vi "update.vi"(8 "error in (no error)":errorcluster, 11 "HSDIO in":refnum<class "HSDIO.lvclass">) -> (0 "error out":errorcluster, 3 "HSDIO out":refnum<class "HSDIO.lvclass">)   [LabVIEW 2013, in "HSDIO.lvclass"]
uses:
  HSDIO.lvclass
  waveform.ctl
  HSDIO.lvclass/HSDIO.ctl
  Globals.vi
  <instrlib>/niHSDIO/niHSDIO.llb/niHSDIO Write Named Waveform (WDT).vi
panel:
  out "transitions":u32[](array[numeric])
  out "states":u8[][](array[numeric])
  out "output waveform":digitaldata
  out "HSDIO Settings.Array of Waveforms":T1[](array[typedef])
  out "HSDIO Settings.Pulse Generation Script":string
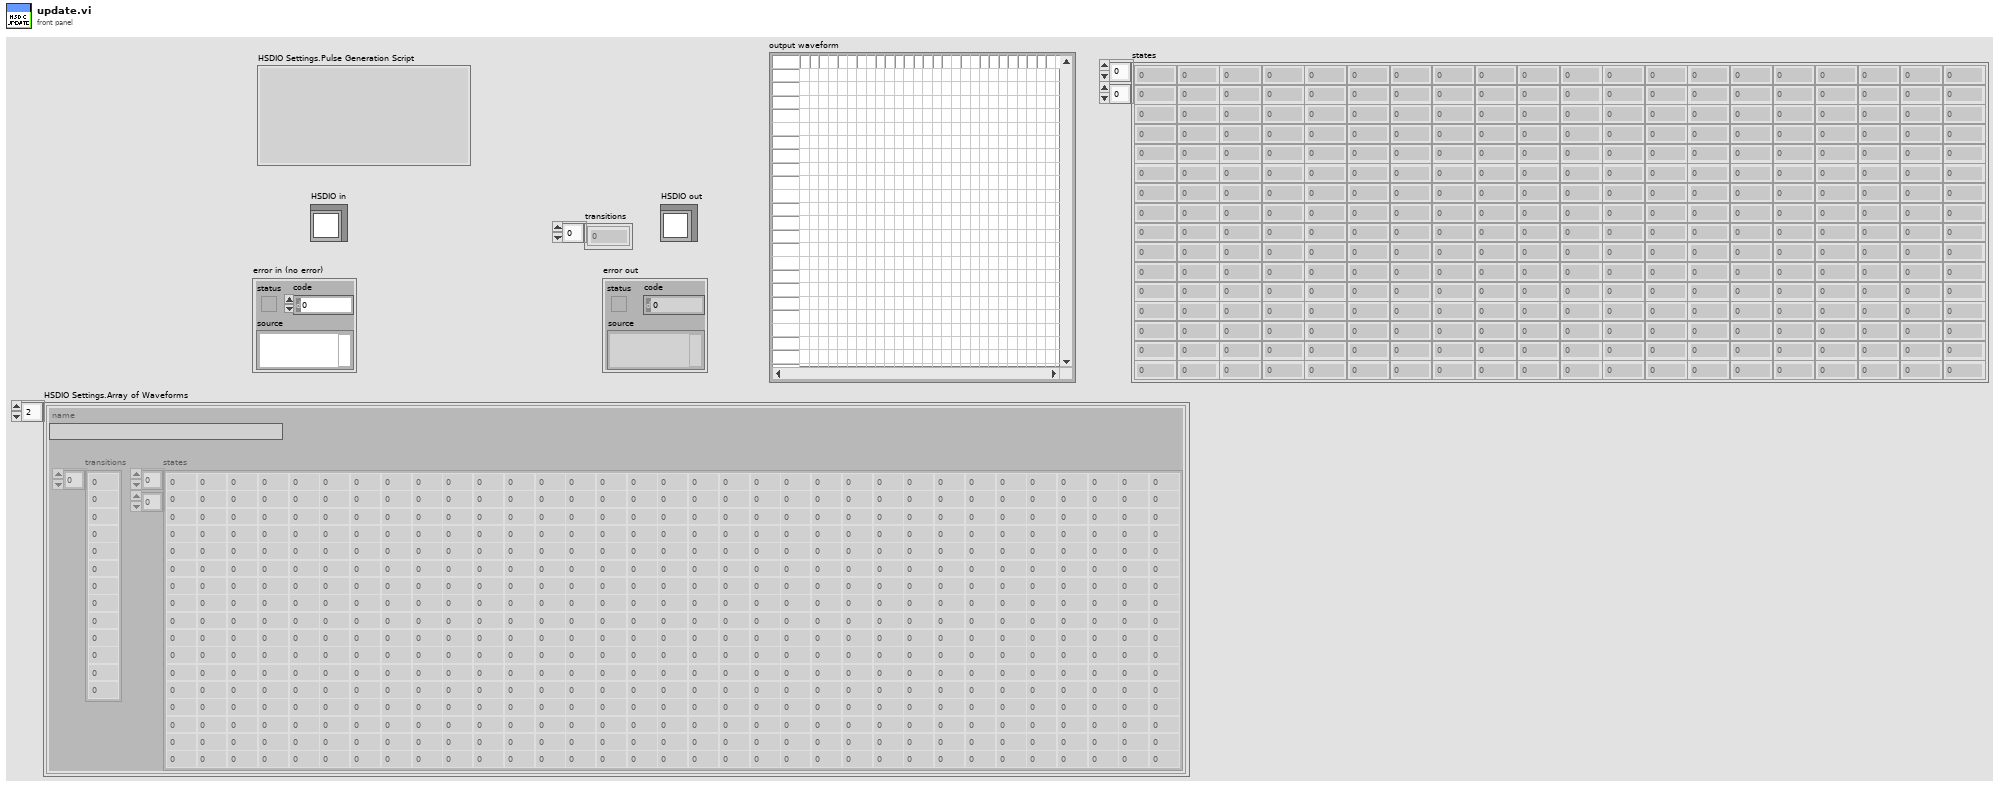
[diagram p1: front panel]
types:
  T1 = typedef "HSDIO.lvclass/waveform.ctl" = cluster{"name":string, "transitions":u32[], "states":u8[][]}
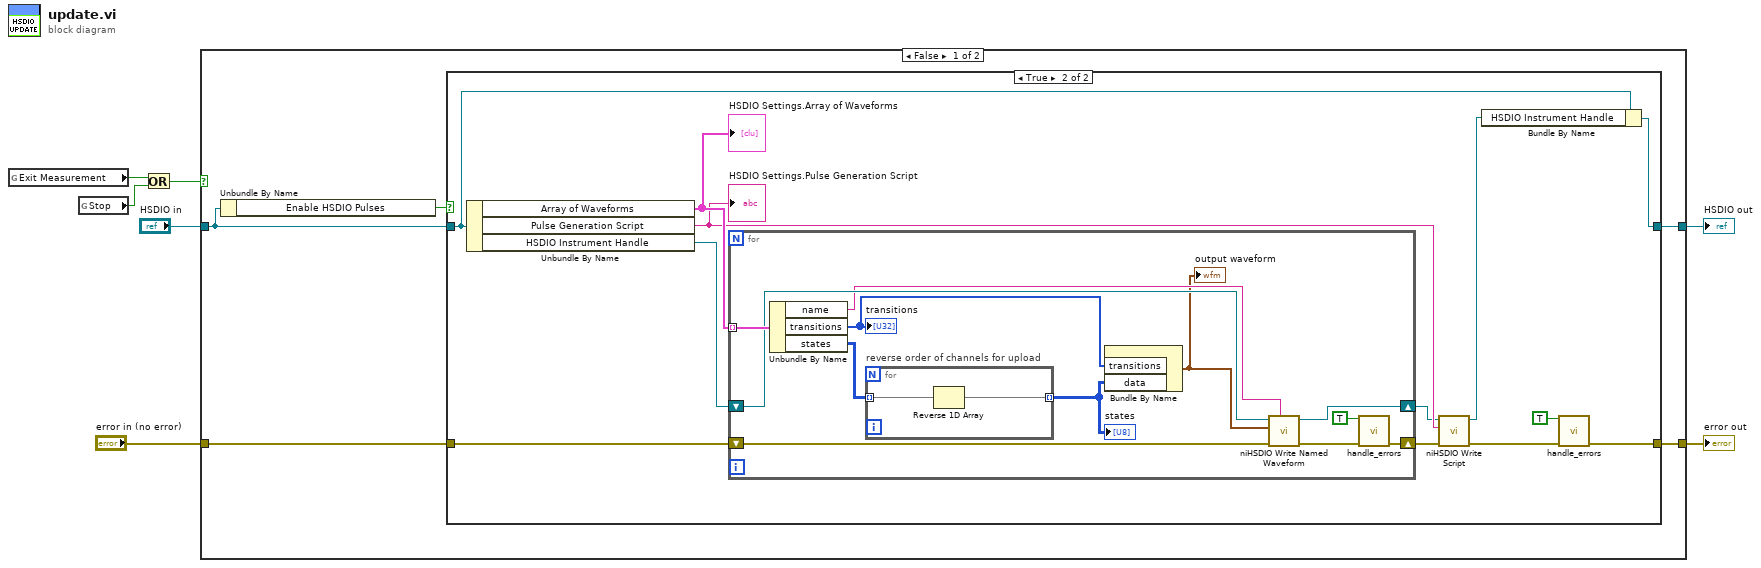
[diagram p0: block diagram]
diagram:
  n1 = global read "Globals.vi" "Exit Measurement"() -> (w3:bool)
  n2 = global read "Globals.vi" "Stop"() -> (w2:bool)
  n3 = Or(x=w3, y=w2) -> (x .or. y?=w1:bool)
  n4 = case shown="False" w1 {
    tunnel: [w8 w41] -> w5
    tunnel: [w10 w42] -> w6
    tunnel: "HSDIO in" -> [w11 w42]
    tunnel: "error in (no error)" -> [w9 w41]
    frame False {
      n5 = Unbundle By Name(w11) -> ("Enable HSDIO Pulses"=w12:bool)
      n6 = case shown="True" w12 {
        tunnel: w11 -> [w14 w24]
        tunnel: [w14 w25] -> w10
        tunnel: w9 -> [w13 w18]
        tunnel: [w13 w16] -> w8
        frame False {
        }
        frame True {
          n7 = Unbundle By Name(w24) -> ("Array of Waveforms"=w23:T1[], "Pulse Generation Script"=w22:string, "HSDIO Instrument Handle"=w21:refnum<k15>)
          "HSDIO Settings.Pulse Generation Script" <- w22
          "HSDIO Settings.Array of Waveforms" <- w23
          n8 = for {
            tunnel: w23 -> [w38] mode=indexing
            shift-right: [w32] -> w19
            shift-left: w18 -> [w34]
            shift-right: [w35] -> w20
            shift-left: w21 -> [w36]
            n9 = Unbundle By Name(w38) -> ("name"=w30:string, "transitions"=w37:u32[], "states"=w28:u8[][])
            "transitions" <- w37
            n10 = for "reverse order of channels for upload" {
              tunnel: w28 -> [w40] mode=indexing
              tunnel: [w39] -> w27 mode=indexing
              n11 = Reverse 1D Array(array=w40) -> (reversed array=w39:u8[])
            }
            "states" <- w27
            n12 = Bundle By Name("transitions"=w37, "data"=w27) -> (w29:digitaldata)  [unwired: 1 in]
            "output waveform" <- w29
            n13 = call-poly <instrlib>:"niHSDIO Write Named Waveform.vi"("waveform name (default:\"\")"=w30, "error in (no error)"=w34, "data"=w29, "instrument handle"=w36) -> ("error out"=w33:errorcluster, "instrument handle out"=w35:refnum<k15>)  [unwired: 6 in]
            n14 = call "handle_errors.vi"("Exit Operation"=TRUE ("Exit Measurement"), "error in (no error)"=w33) -> ("error out"=w32:errorcluster)  [unwired: 13 in]
          }
          n15 = call <instrlib>:"niHSDIO Write Script.vi"("error in (no error)"=w19, "script"=w22, "instrument handle"=w20) -> ("error out"=w17:errorcluster, "instrument handle out"=w26:refnum<k15>)  [unwired: 7 in]
          n16 = Bundle By Name(cluster=w24, "HSDIO Instrument Handle"=w26) -> (w25:refnum<class "HSDIO.lvclass">)
          n17 = call "handle_errors.vi"("Exit Operation"=TRUE ("Exit Measurement"), "error in (no error)"=w17) -> ("error out"=w16:errorcluster)  [unwired: 13 in]
        }
      }
    }
    frame True {
    }
  }
  "error out" <- w5
  "HSDIO out" <- w6
